vi "monochromator_cmd.vi"(8 "error in (no error)":errorcluster, 9 "Parameter":string, 10 "Command":string(combo), 11 "Addr in":string="ASRL5::INSTR") -> (0 "error out":errorcluster, 1 "standard error":string, 2 "standard output":string, 3 "Addr out":string)   [LabVIEW 2018]
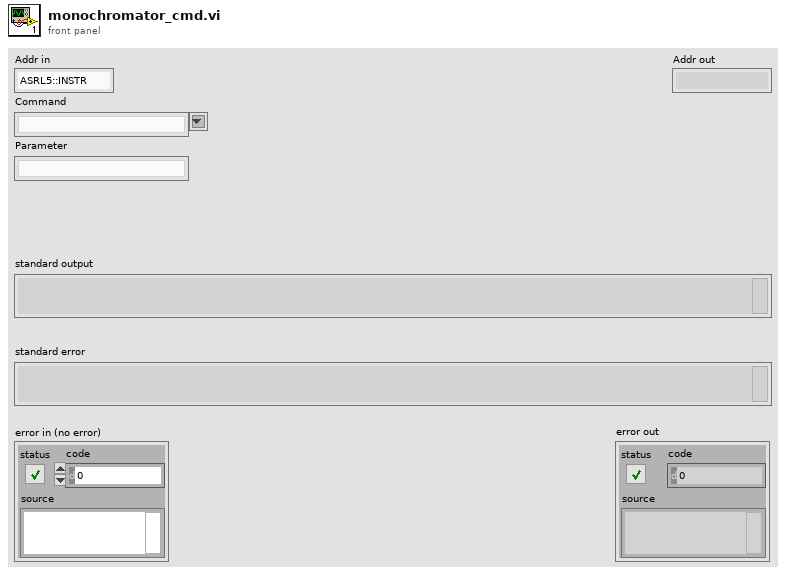
[diagram p1: front panel]
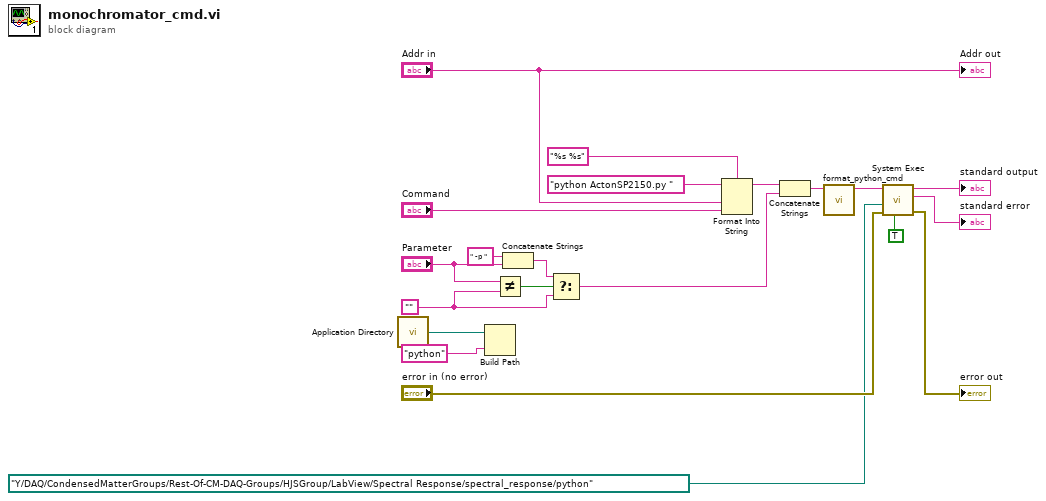
[diagram p0: block diagram]
diagram:
  w10 = ""
  n1 = call <vilib>:"Application Directory.vi"() -> ("Application Directory"=w18:path)
  n2 = Build Path(base path=w18, name or relative path="python") -> ()  [unwired: 1 out]
  n3 = Not Equal?(x="Parameter", y=w10) -> (x != y?=w14:bool)
  n4 = Concatenate Strings(" -p " ("string"), "Parameter") -> (w11:string)
  n5 = Select(t=w11, s=w14, f=w10) -> (s? t:f=w9:string)
  n6 = Format Into String(format string="%s %s", initial string="python ActonSP2150.py ", "Addr in", "Command") -> (resulting string=w15:string)  [unwired: 1 in, 1 out]
  n7 = Concatenate Strings(w15, w9) -> (w8:string)
  n8 = call "format_python_cmd.vi"("python cmd"=w8) -> ("system exec python cmd"=w7:string)  [unwired: 10 in]
  n9 = call <vilib>:"System Exec.vi"("run minimized? (F)"=TRUE, "error in (no error)"="error in (no error)", "working directory"=path "Y:/DAQ/CondensedMatterGroups/Rest-Of-CM-DAQ-Groups/HJSGroup/LabView/Spectral Response/spectral_response/python", "command line"=w7) -> ("error out"=→"error out":errorcluster, "standard error"=→"standard error":string, "standard output"=→"standard output":string)  [unwired: 4 in, 1 out]
  "Addr out" <- "Addr in"
